vi "Meel2Freq(1D).vi"(11 "Mel":dbl[](array[numeric])) -> (3 "Freq":dbl[](array[numeric]))   [LabVIEW 2020]
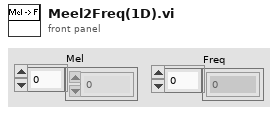
[diagram p1: front panel]
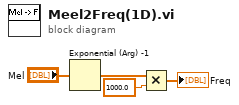
[diagram p0: block diagram]
diagram:
  n1 = Exponential (Arg) -1(1:"Mel") -> (0:w1:dbl[])
  n2 = Multiply(x=w1, y=1000.0) -> (x*y=→"Freq":dbl[])
